vi "Read Tab Into.vi"(9 "Tab in":refnum<class "Tab.lvclass">) -> (3 "Tab out":refnum<class "Tab.lvclass">, 4 "Tab Into":bool)   [LabVIEW 2014, in "Raspberry Pi Compatible Compiler for LabVIEW.lvlib" / "Tab.lvclass"]
uses:
  Tab.lvclass
  Tab.lvclass/Tab.ctl
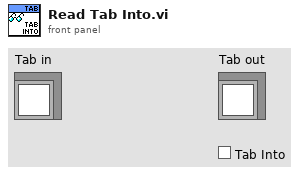
[diagram p1: front panel]
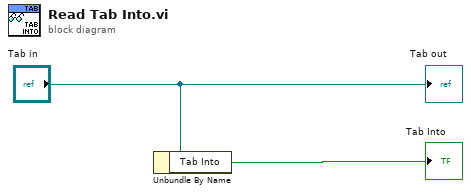
[diagram p0: block diagram]
diagram:
  n1 = Unbundle By Name("Tab in") -> ("Tab Into"=→"Tab Into":bool)
  "Tab out" <- "Tab in"
